vi "Create TCP Stream Listener.vi"(9 "Local Port":u16) -> (3 "TCP Stream Listener":refnum<class "TCP Stream Listener.lvclass">)   [LabVIEW 2020, in "TCP Stream Listener.lvclass"]
doc: "Use this method to configure a TCP Stream Listener with the local port it will use."
uses:
  TCP Stream Listener.lvclass
  TCP Stream/TCP Stream.lvclass
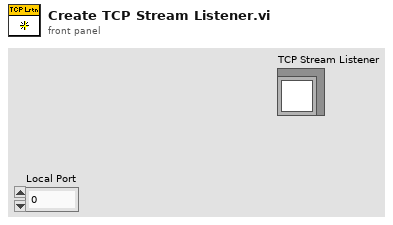
[diagram p1: front panel]
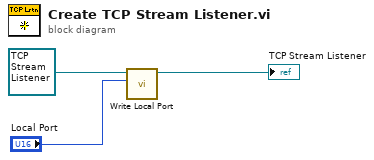
[diagram p0: block diagram]
diagram:
  n1 = call "Write Local Port.vi"("local port"="Local Port", "TCP Stream in"=refnum<class "TCP Stream Listener.lvclass"> refnum ("TCP Stream Listener.lvclass")) -> ("TCP Stream out"=→"TCP Stream Listener":refnum<class "TCP Stream Listener.lvclass">)  [unwired: 9 in]
